vi "Exit the DAQ Engine.vi"   [LabVIEW 2009]
uses:
  Controls/SLL DE DAQ Global Options.ctl
  Controls/SLL DE DAQ Global Elements.ctl
types:
  T1 = typedef "SLL DE DAQ Global Options.ctl" = enum16{"Init", "Write 1", "Read 1", "Write Array", "Read Array", "Clear"}
  T2 = typedef "SLL DE DAQ Global Elements.ctl" = enum16{"AI Error", "AO Error", "DI Error", "DO Error", "AI Restart", "DI Restart", "AI Running", "AO Running", "DI Running", "DO Running", "DAQ Exit?"}
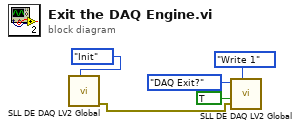
[diagram p0: block diagram]
diagram:
  n1 = call "SLL DE DAQ LV2 Global.vi"("Option"=SLL_DE_DAQ_Global_Options."Init") -> ("error out"=w1:errorcluster)  [unwired: 8 in, 2 out]
  n2 = call "SLL DE DAQ LV2 Global.vi"("Option"=SLL_DE_DAQ_Global_Options."Write 1", "error in (no error)"=w1, "Status In"=TRUE, "Element"=SLL_DE_DAQ_Global_Elements."DAQ Exit?") -> ()  [unwired: 5 in, 3 out]
